vi "hmi_halo_drive.vi"(10 "Wheel":dbl, 11 "Throttle":dbl) -> (3 "Drive Data":cluster{"Left":dbl, "Right":dbl})   [LabVIEW 2011]
panel:
  in  "QuickTurn Const":dbl=0.25
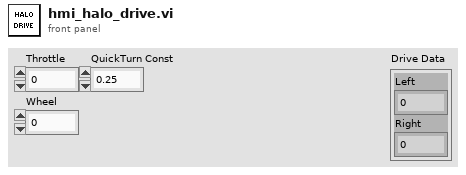
[diagram p1: front panel]
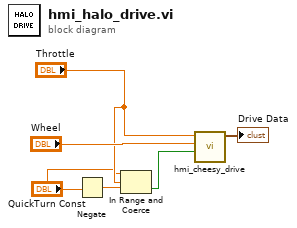
[diagram p0: block diagram]
diagram:
  n1 = Negate(x="QuickTurn Const") -> (-x=w3:dbl)
  n2 = In Range and Coerce(upper limit="QuickTurn Const", x="Throttle", lower limit=w3) -> (In Range?=w1:bool)  [unwired: 1 out]
  n3 = call "hmi_cheesy_drive.vi"("Quick Turn"=w1, "Wheel"="Wheel", "Throttle"="Throttle") -> ("Drive Data"=→"Drive Data":cluster{"Left":dbl, "Right":dbl})  [unwired: 8 in]
